vi "DriftFileHeader(SubVI).vi"(0 "Start value (V)":sgl, 1 "Byte Stream File in":refnum<file>, 3 "Drift Correction":T1={"Drift correction Pixels"=256, "Imaging Current"=1.5e-11, "STS Current"=1.15e-09, "MaxImagesBack"=40, "tip Speed (m/s)"=1e-08, "Threshold"=2, "Increment"=40, "Correlate"=0, "max applied Drift Correction"=20, "Imaging Bias"=-0.01, "Move Current"=1.5e-11, "Move Bias"=-0.01, "STS Bias"=0.005, "preSTS delay [ms]"=3, "STS z offset"=1.15e-09, "Correct Drift"=FALSE, "Lockin ON/OFF"=FALSE} {"STS z offset" format="%#_6p"; "STS Bias" format="%#_6p"; "Move Bias" format="%#_6p"; "Move Current" format="%#_6p"; "Imaging Bias" format="%#_6p"; "max applied Drift Correction" min=1 max=100 step=1 format="%.0p"; "Correlate" items=["first Frame", "successive Frames"]; "Threshold" min=1 step=1; "tip Speed (m/s)" format="%.2p"; "STS Current" format="%#_6p"; "Imaging Current" format="%#_6p"}, 5 "End of Sweep":T4, 7 "Application ref in":refnum<vi>, 9 "End value (V)":sgl, 11 "error in (no error)":errorcluster, 12 "Sweep Timing":T2, 14 "Initialization":T3) -> (4 "Byte Stream File out":refnum<file>, 8 "Application ref out":refnum<vi>)   [LabVIEW 2014]
panel:
  # "% of image size"
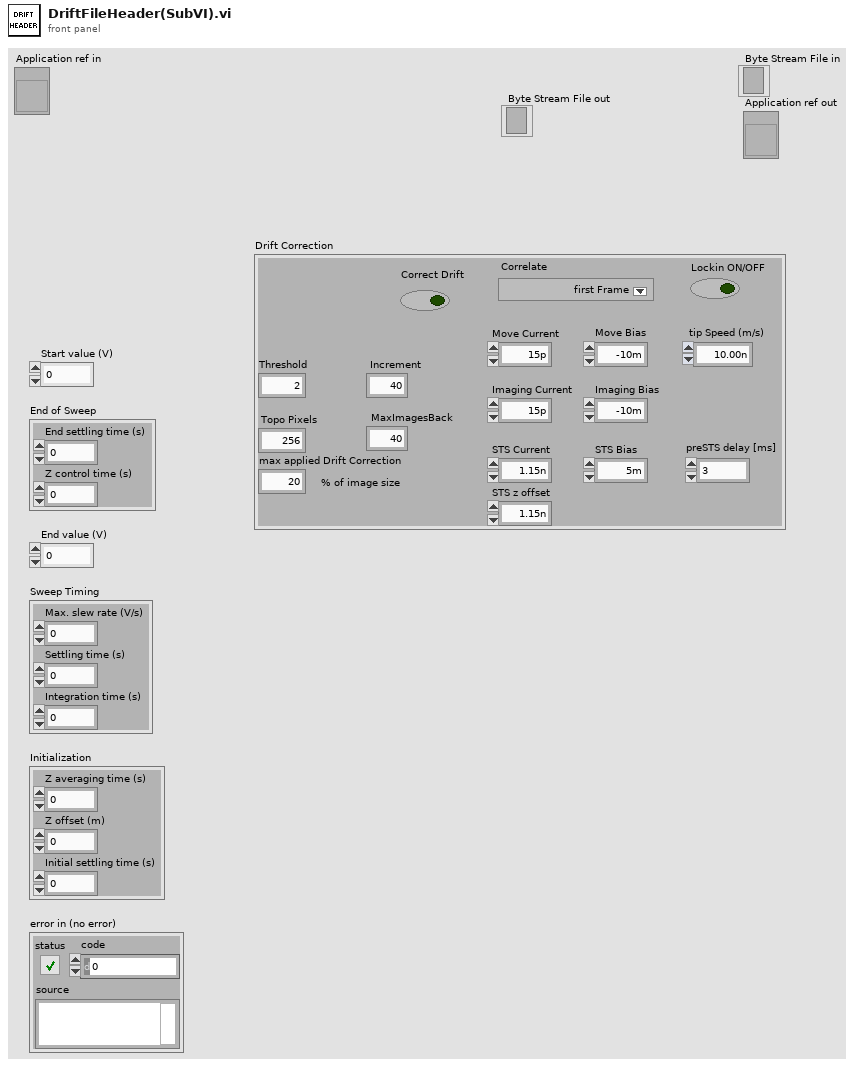
[diagram p1: front panel]
types:
  T1 = cluster{"Drift correction Pixels":i32, "Imaging Current":dbl, "STS Current":dbl, "MaxImagesBack":i32, "tip Speed (m/s)":sgl, "Threshold":i32, "Increment":i32, "Correlate":u16, "max applied Drift Correction":i32, "Imaging Bias":dbl, "Move Current":dbl, "Move Bias":dbl, "STS Bias":dbl, "preSTS delay [ms]":u32, "STS z offset":dbl, "Correct Drift":bool, "Lockin ON/OFF":bool}
  T2 = cluster{"Max. slew rate (V/s)":sgl, "Settling time (s)":sgl, "Integration time (s)":sgl}
  T3 = cluster{"Z averaging time (s)":sgl, "Z offset (m)":sgl, "Initial settling time (s)":sgl}
  T4 = cluster{"End settling time (s)":sgl, "Z control time (s)":sgl}
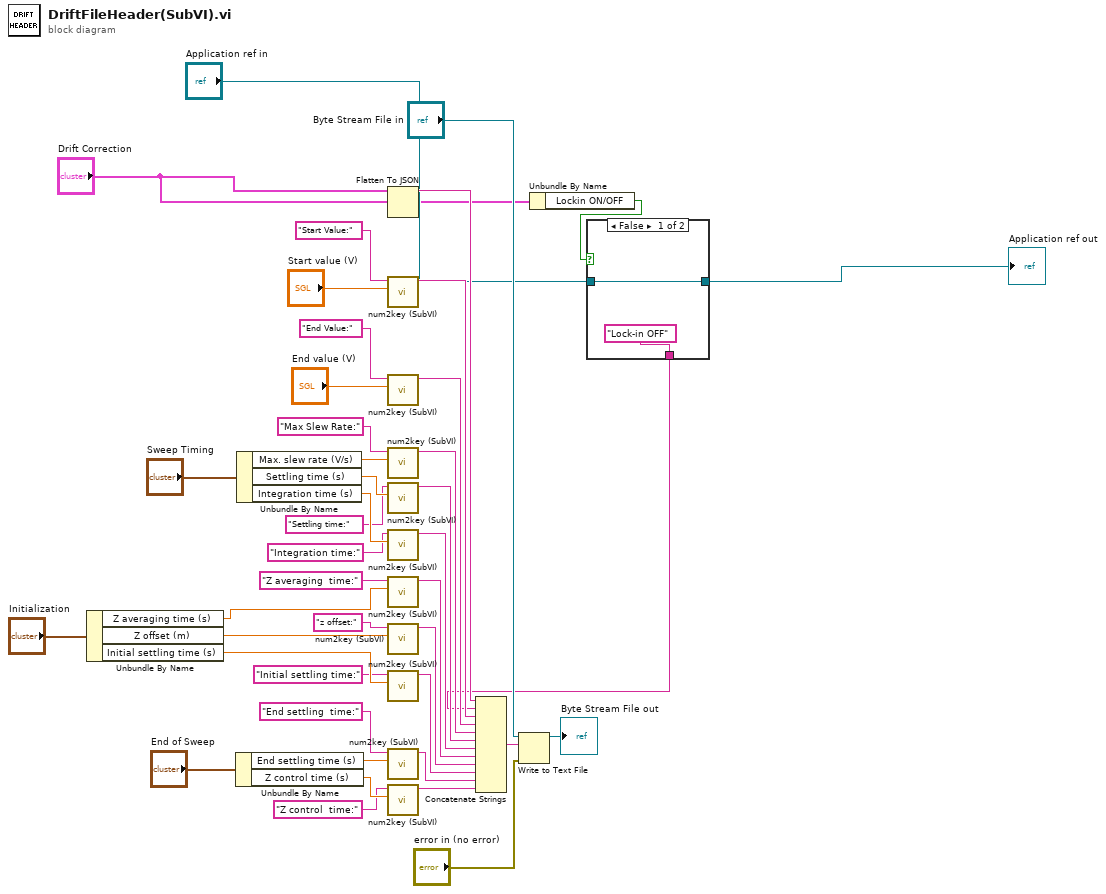
[diagram p0: block diagram]
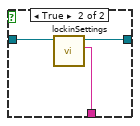
[diagram p2: hidden frame]
diagram:
  n1 = Unbundle By Name("Initialization") -> ("Z averaging time (s)"=w26:sgl, "Z offset (m)"=w25:sgl, "Initial settling time (s)"=w28:sgl)
  n2 = Unbundle By Name("End of Sweep") -> ("End settling time (s)"=w32:sgl, "Z control time (s)"=w31:sgl)
  n3 = Unbundle By Name("Sweep Timing") -> ("Max. slew rate (V/s)"=w18:sgl, "Settling time (s)"=w19:sgl, "Integration time (s)"=w20:sgl)
  n4 = Flatten To JSON(anything="Drift Correction") -> (JSON string=w6:string)  [unwired: 2 in, 1 out]
  n5 = call "num2key (SubVI).vi"("Img current"="Start value (V)", "String in"="Start Value:") -> ("String out"=w33:string)  [unwired: 9 in]
  n6 = call "num2key (SubVI).vi"("Img current"="End value (V)", "String in"="End Value:") -> ("String out"=w34:string)  [unwired: 9 in]
  n7 = call "num2key (SubVI).vi"("Img current"=w18, "String in"="Max Slew Rate:") -> ("String out"=w35:string)  [unwired: 9 in]
  n8 = call "num2key (SubVI).vi"("Img current"=w19, "String in"="Settling time:") -> ("String out"=w36:string)  [unwired: 9 in]
  n9 = call "num2key (SubVI).vi"("Img current"=w20, "String in"="Integration time:") -> ("String out"=w37:string)  [unwired: 9 in]
  n10 = call "num2key (SubVI).vi"("Img current"=w26, "String in"="Z averaging  time:") -> ("String out"=w38:string)  [unwired: 9 in]
  n11 = call "num2key (SubVI).vi"("Img current"=w25, "String in"="z offset:") -> ("String out"=w39:string)  [unwired: 9 in]
  n12 = call "num2key (SubVI).vi"("Img current"=w28, "String in"="Initial settling time:") -> ("String out"=w40:string)  [unwired: 9 in]
  n13 = call "num2key (SubVI).vi"("Img current"=w32, "String in"="End settling  time:") -> ("String out"=w41:string)  [unwired: 9 in]
  n14 = call "num2key (SubVI).vi"("Img current"=w31, "String in"="Z control  time:") -> ("String out"=w42:string)  [unwired: 9 in]
  n15 = Unbundle By Name("Drift Correction") -> ("Lockin ON/OFF"=w2:bool)
  n16 = case shown="False" w2 {
    tunnel: "Application ref in" -> [w45 w48]
    tunnel: [w45 w47] -> w4
    tunnel: ["Lock-in OFF" ("concatenated string") w46] -> w1
    frame False {
    }
    frame True {
      n17 = call "lockinSettings.vi"("Application ref in"=w48) -> ("concatenated string"=w46:string, "Application ref out"=w47:refnum<vi>)  [unwired: 6 in, 1 out]
    }
  }
  "Application ref out" <- w4
  n18 = Concatenate Strings(w6, w1, w33, w34, w35, w36, w37, w38, w39, w40, w41, w42) -> (w43:string)
  n19 = Write to Text File(file (use dialog)="Byte Stream File in", text=w43, error in="error in (no error)") -> (refnum out=→"Byte Stream File out":refnum<file>)  [unwired: 1 in, 2 out]
